vi "connectToRemoteMachine.vi"(8 "error in (no error)":errorcluster, 9 "remote port":u16, 10 "remote address":string, 11 "NetworkServer in":refnum<class "NetworkServer.lvclass">) -> (0 "error out":errorcluster, 3 "NetworkServer out":refnum<class "NetworkServer.lvclass">)   [LabVIEW 2009, in "Hardware.lvlib" / "HWControllers.lvlib" / "NetworkServer.lvclass"]
uses:
  NetworkServer.lvclass
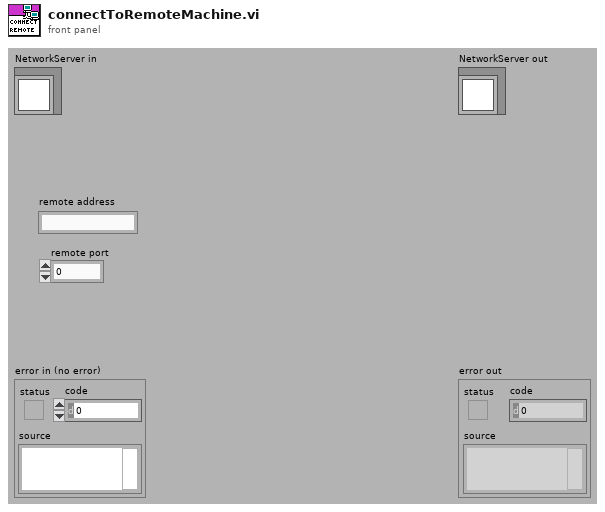
[diagram p1: front panel]
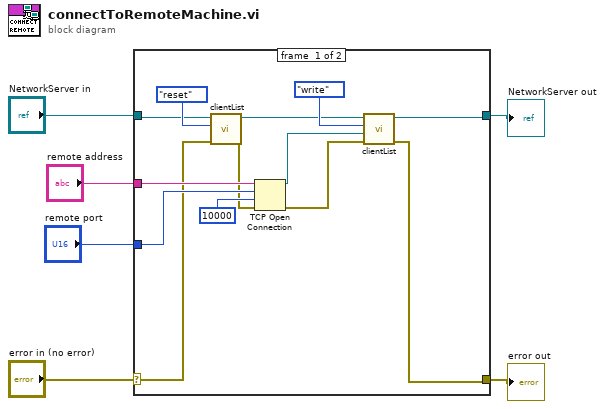
[diagram p0: block diagram]
diagram:
  n1 = case shown="No Error" "error in (no error)" {
    selector: "error in (no error)" -> [w7 w21]
    tunnel: [w13 w21] -> w5
    tunnel: [w12 w20] -> w3
    tunnel: "NetworkServer in" -> [w10 w20]
    tunnel: "remote address" -> [w19 _]
    tunnel: "remote port" -> [w18 _]
    frame #0 {
      n2 = call "clientList.vi"("error in (no error)"=w7, "Enum"=enum16{"read", "write", "reset"}."reset", "NetworkServer in"=w10) -> ("error out"=w8:errorcluster, "NetworkServer out"=w9:refnum<class "NetworkServer.lvclass">)  [unwired: 5 in, 2 out]
      n3 = TCP Open Connection(address=w19, remote port or service name=w18, timeout ms (60000)=10000, error in (no error)=w8) -> (connection ID=w16:refnum<k5>, error out=w14:errorcluster)  [unwired: 1 in]
      n4 = call "clientList.vi"("error in (no error)"=w14, "new client"=w16, "Enum"=enum16{"read", "write", "reset"}."write", "NetworkServer in"=w9) -> ("error out"=w13:errorcluster, "NetworkServer out"=w12:refnum<class "NetworkServer.lvclass">)  [unwired: 4 in, 2 out]
    }
    frame #1 {
    }
  }
  "error out" <- w5
  "NetworkServer out" <- w3
